vi "CALC_MARK_BWID.vi"(0 "VISA IN":refnum<visa-resource-name>, 1 "Filter Peak":i32, 5 "error in":errorcluster, 7 "Channel":i32) -> (14 "VISA Out":refnum<visa-resource-name>, 19 "error out":errorcluster)   [LabVIEW 2018, in "PNA-X.lvlib"]
doc: "CALCulate<cnum>:MARKer:BWIDth <num> \n(Read-Write) Turns on and sets markers 1 through 4 to calculate filter bandwidth. The <num> \nparameter sets the value below the maximum bandwidth peak that establishes the bandwidth of a \nfilter. For example, if you want to determine the filter bandwidth 3 db below the bandpass peak value, \nset <num> to -3. \nThis feature activates markers 1 through 4. To turn off these markers, either turn them off individually \nor turn them All Off. \nThe analyzer screen will show either Bandwidth statistics OR Trace statistics; not both. \nTo search a User Range with the bandwidth search, first activate marker 1 and set the desired User \nRange. Then send the CALC:MARK:BWID command. The user range used with bandwidth search \nonly applies to marker 1 searching for the max value. The other markers may fall outside the user \nrange. \nSee Critical Note \nParameters \n<cnum> Channel number of the measurement. There must be a selected measurement \non that channel. If unspecified, <cnum> is set to 1. \n<num> Target value below filter peak. Choose any number between :-500 and 500 \nExamples CALC:MARK:BWID -3 \ncalculate2:marker:bwidth -2.513 \nQuery Syntax CALCulate<cnum>:MARKer:BWIDth? \nReturns the results of bandwith search: \n1528\n\nReturn Type Numeric - Four Character values separated by commas: bandwidth, center \nFrequency, Q, loss. \nDefault -3"
uses:
  PNA-X.lvlib
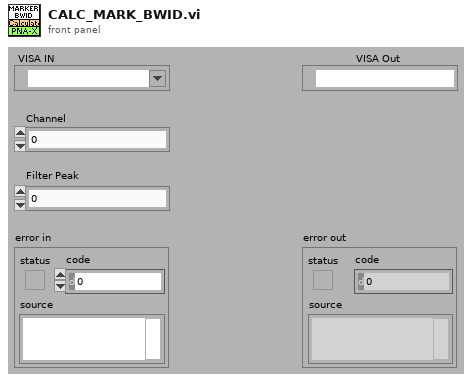
[diagram p1: front panel]
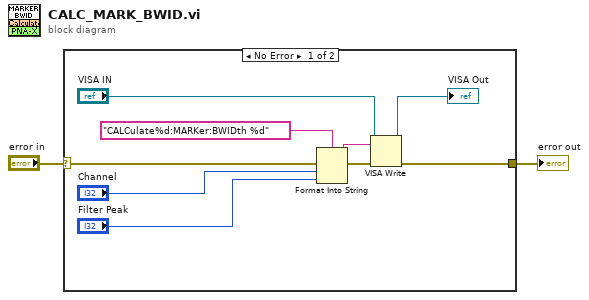
[diagram p0: block diagram]
diagram:
  n1 = case shown="No Error" "error in" {
    selector: "error in" -> [w11 w12]
    tunnel: [w6 w12] -> w1
    frame No Error {
      n2 = Format Into String(format string="CALCulate%d:MARKer:BWIDth %d" ("Cmdline"), error in=w11, "Channel", "Filter Peak") -> (resulting string=w9:string, error out=w10:errorcluster)  [unwired: 1 in]
      n3 = VISA Write(VISA resource name="VISA IN", write buffer=w9, error in (no error)=w10) -> (VISA resource name out=→"VISA Out":refnum<visa-resource-name>, error out=w6:errorcluster)  [unwired: 1 out]
    }
    frame Error {
    }
  }
  "error out" <- w1
